vi "Build version and date.vi"(8 "error in":errorcluster) -> (0 "error out":errorcluster, 1 "Development?":bool, 2 "Build date":string, 3 "Revision":i32)   [LabVIEW 2013]
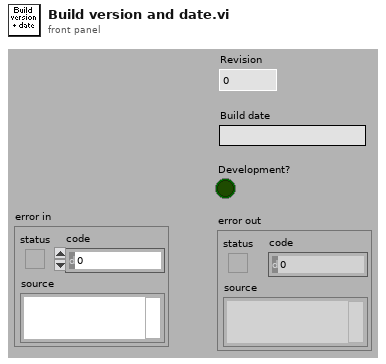
[diagram p1: front panel]
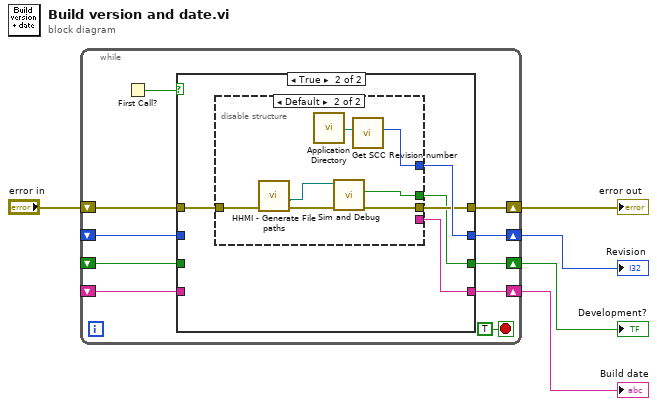
[diagram p0: block diagram]
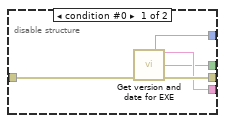
[diagram p3: hidden frame]
diagram:
  n1 = while {
    shift-right: [w13] -> w3
    shift-left: _ -> [w9]
    shift-right: [w15] -> w5
    shift-left: _ -> [w8]
    shift-right: [w12] -> w2
    shift-left: _ -> [w10]
    shift-right: [w7] -> w1
    shift-left: "error in" -> [w14]
    stop <- TRUE stop-if-true
    n2 = First Call?() -> (First Call?: T/F=w11:bool)
    n3 = case shown="True" w11 {
      tunnel: [w17 w24] -> w15
      tunnel: w14 -> [w16 w23]
      tunnel: [w18 w22] -> w13
      tunnel: [w16 w21] -> w7
      tunnel: [w19 w20] -> w12
      tunnel: w10 -> [w19 _]
      tunnel: w9 -> [w18 _]
      tunnel: w8 -> [w17 _]
      frame False {
      }
      frame True {
        n4 = disable-structure shown="Default" {
          disable-tunnel: [w29 w33] -> w22
          disable-tunnel: [w28 w36] -> w21
          disable-tunnel: w23 -> [w27 w32]
          disable-tunnel: [w26 _] -> w24
          disable-tunnel: [w25 w35] -> w20
          frame condition #0 {
            n5 = call "Get version and date for EXE.vi"("error out"=w27) -> ("Version"=w29:i32, "Build date"=w26:string, "Development Version?"=w25:bool, "error out"=w28:errorcluster)  [unwired: 10 in, 1 out]
          }
          frame condition #1 (active) {
            n6 = call "HHMI - Generate File paths.vi"("error in"=w32) -> ("error out"=w30:errorcluster, "Project path"=w31:path)  [unwired: 8 in, 1 out]
            n7 = call <vilib>:"Application Directory.vi"() -> ("Application Directory"=w34:path)
            n8 = call "Sim and Debug.vi"("error in"=w30, "Path"=w31) -> ("error out"=w36:errorcluster, "Development?"=w35:bool)  [unwired: 6 in, 2 out]
            n9 = call "Get SCC Revision number.vi"("path"=w34) -> ("Revision"=w33:i32)  [unwired: 10 in]
          }
        }
      }
    }
  }
  "Build date" <- w5
  "Revision" <- w3
  "error out" <- w1
  "Development?" <- w2
